vi "OpenUDP.vi"(8 "错误输入（无错误）":errorcluster, 9 "本地端口":u16=65502, 10 "目的端口":u16=65502, 11 "目的IP地址":string="192.168.3.39") -> (0 "错误输出":errorcluster, 3 "连接输出":T1)   [LabVIEW 2018]
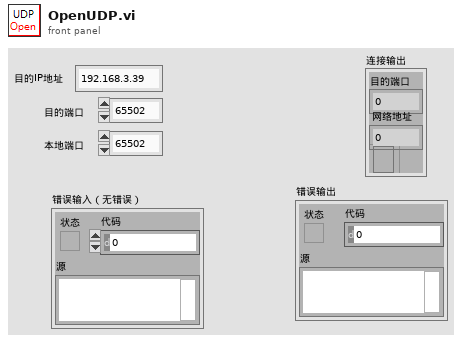
[diagram p1: front panel]
types:
  T1 = cluster{"目的端口":u16, "网络地址":u32, "连接ID":refnum<k16>}
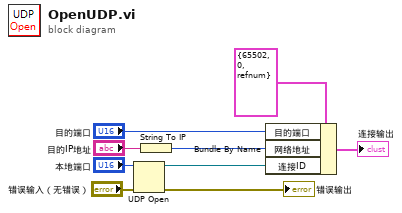
[diagram p0: block diagram]
diagram:
  n1 = UDP Open(8:"错误输入（无错误）", 11:"本地端口") -> (port=w2:refnum<k16>, 0:→"错误输出":errorcluster)  [unwired: 3 in, 1 out]
  n2 = String To IP(1:"目的IP地址") -> (0:w4:u32)
  n3 = Bundle By Name(cluster=T1 {"目的端口"=65502, "网络地址"=0, "连接ID"=refnum} ("连接"), "目的端口"="目的端口", "网络地址"=w4, "连接ID"=w2) -> (→"连接输出":T1)
